vi "cRio_JKS_v5.vi"() -> ()   [LabVIEW 2017]
uses:
  <vilib>/LabVIEW Targets/FPGA/cRIO/shared/nicrio_ModuleControls/nicrio_cRIO-9237_ExcitationVoltageRing.ctl
  <vilib>/LabVIEW Targets/FPGA/cRIO/shared/nicrio_ModuleControls/nicrio_cRIO-9237_DataRatesRing.ctl
  <vilib>/Platform/TimedLoop/XDataNode/timing_clust.ctl
  <vilib>/Platform/TimedLoop/XDataNode/nitl_modes.ctl
  <vilib>/Platform/TimedLoop/XDataNode/wakeup.ctl
  <vilib>/Analysis/3filter.llb/Filter Passband Type.ctl
  <vilib>/rvi/Analysis/host/Butterworth/config/Butterworth Filter Order.ctl
  <vilib>/rvi/Analysis/host/Butterworth/config/Butterworth Filter Type.ctl
  <vilib>/Simulation/Scripting/Companion Diagram/SimConfigNode/SimParams.ctl
  <vilib>/Simulation/Scripting/Companion Diagram/SimConfigNode/_simSolvers.ctl
  <vilib>/Simulation/Implementation/Shared/SIMSCR Execution Mode.ctl
  <vilib>/Simulation/Param Hierarchy/Typedefs/SIMPH Param Control Actions.ctl
  <vilib>/Simulation/Implementation/Shared/NILVSim_ParamChanged.vi
  <vilib>/Simulation/Implementation/Shared/NILVSIM_BeginStep.vi
  <vilib>/Simulation/Implementation/Shared/NILVSim_Manager.vi
  <vilib>/Utility/error.llb/Clear Errors.vi
  <vilib>/Simulation/Implementation/Shared/NILVSim_FinalizeModel.vi
  <vilib>/FPGAPlugInAG/cRIO-9111/niLvFpga_Open_cRIO-9111.vi
  <vilib>/rvi/interface/common/dynamic/niFpgaDynamicAddResources.vi
  <vilib>/rvi/Analysis/host/Butterworth/config/BwScaledCoefficients.vi
  <vilib>/Utility/error.llb/Error Cluster From Error Code.vi
  <vilib>/rvi/errors/niLvFpgaAdjustHostInterfaceError.vi
  <vilib>/Simulation/Implementation/Shared/SIM Unbundle Sim Info.vi
  <vilib>/Simulation/Implementation/Shared/NILVSim_Initialize.vi
  <vilib>/Simulation/Utility/Implementation/NILVSim Get Time and IsAcceptedStep.vi
  <vilib>/Simulation/Implementation/Shared/SIMSH Read Queue.vi
  <vilib>/Simulation/Implementation/Shared/NILVSim_GetModelError.vi
  <vilib>/Simulation/Implementation/Shared/SIM Bundle Sim Info.vi
  <vilib>/FPGAPlugInAG/Dynamic/niLvFpga_Close_Dynamic.vi
  <vilib>/Platform/TimedLoop/XDataNode/XDataNode.xnode
  <vilib>/rvi/interface/nirviOpenFPGA/nirviOpenFPGA.xnode
  FPGA Bitfiles/testrigv1_FPGATarget2_FPGAv3_Z7WGzOqu7JU.lvbitx
  FPGA_JKS_v1.vi
  <vilib>/rvi/Analysis/host/Butterworth/XNode/ButterworthCoefficients.xnode
  <vilib>/rvi/interface/nirviReadWriteControl/nirviReadWriteControl.xnode
  <vilib>/Simulation/Implementation/XNodeFramework/SimXNode/SimX.xnode
  PID (Parallel) with monitoring.vi
  <vilib>/Simulation/Scripting/Companion Diagram/SimConfigNode/SimDog.xnode
  <vilib>/rvi/interface/nirviCloseFPGA/nirviCloseFPGA.xnode
  <vilib>/Platform/TimedLoop/XDataNode/XDNodeRunTimeDep.lvlib
  <vilib>/rvi/interface/Simulation/niFpgaSimulationCallBeginRW.vi
  <vilib>/rvi/Analysis/host/Public/NI_FpgaMspHost.lvlib
  <vilib>/Analysis/NI_AALBase.lvlib
  <vilib>/ptbypt/NI_PtbyPt.lvlib
  NiFpgaLv.dll
  <vilib>/Simulation/Implementation/Shared/NI_SIM_Implementation.lvlib
panel:
  in  "Data Rate Strain Gauge":T1=1 items=["50.000 kS/s (NI 9237)"=1, "25.000 kS/s (NI 9237)"=2, "16.667 kS/s (NI 9237)"=3, "12.500 kS/s (NI 9237)"=4, "10.000 kS/s (NI 9237)"=5, "8.333 kS/s (NI 9237)"=6, "7.143 kS/s (NI 9237)"=7, "6.250 kS/s (NI 9237)"=8, "5.556 kS/s (NI 9237)"=9, "5.000 kS/s (NI 9237)"=10, "4.545 kS/s (NI 9237)"=11, "4.167 kS/s (NI 9237)"=12, "3.846 kS/s (NI 9237)"=13, "3.571 kS/s (NI 9237)"=14, "3.333 kS/s (NI 9237)"=15, "3.125 kS/s (NI 9237)"=16, "2.941 kS/s (NI 9237)"=17, "2.778 kS/s (NI 9237)"=18, "2.632 kS/s (NI 9237)"=19, "2.500 kS/s (NI 9237)"=20, "2.381 kS/s (NI 9237)"=21, "2.273 kS/s (NI 9237)"=22, "2.174 kS/s (NI 9237)"=23, "2.083 kS/s (NI 9237)"=24, "2.000 kS/s (NI 9237)"=25, "1.923 kS/s (NI 9237)"=26, "1.852 kS/s (NI 9237)"=27, "1.786 kS/s (NI 9237)"=28, "1.724 kS/s (NI 9237)"=29, "1.667 kS/s (NI 9237)"=30, "1.613 kS/s (NI 9237)"=31]
  in  "Excitation Voltage Strain Gauge":T2 items=["2.5 Volts", "3.3 Volts", "5.0 Volts", "10.0 Volts", "External Excitation"]
  in  "dpOpen (bar)":sgl=1.0
  out "Run_time slow":dbl
  out "actual_FPGA_dt_(uSec)":u32=50
  out "Actual loop time (mSec)":u32=10
  out "Active.log":bool
  in  "Start.log":bool
  out "P.B.HP":dbl format="%0.2f"
  out "P.B":dbl
  out "P.A1":dbl
  out "P.A":dbl
  out "P.comp":dbl
  out "P.return":dbl
  out "P.pump":dbl
  out "Q.B":dbl format="%0.2f"
  out "FB.Bosch":dbl format="%0.2f"
  out "FB.DCV":dbl format="%0.2f"
  out "u_Bosch":dbl
  out "x.c":dbl
  out "P.B.LP":dbl format="%0.2f"
  out "x.c.dot":dbl
  out "dLcyl filtered":dbl format="%0.2f"
  out "dt":dbl
  in  "Tab Control":enum32{"Settings", "DCV", "Bosch", "ROD"}(tab)
  in  "Bosch mapping 200bar - opening based":cluster{dbl, dbl}[](array[cluster])=[{7.0, 0.0103}, {11.2, 0.032}, {22.0, 0.0535}, {37.0, 0.087}, {61.0, 0.187}, {78.0, 0.289}]
  out "tau (dL)":dbl
  in  "offset_Q_B[V]":sgl=-0.0121
  out "tau (P.B.HP)":dbl
  out "tau (P.B.LP)":dbl
  out "Actual loop time (mSec) slow":u32=10
  in  "Loop time high priority[ms]":i64=10
  in  "cutoff frequency (Hz) FB_Hawe":dbl=300.0
  in  "sample rate (S/s) FB_Hawe":dbl=50000.0
  in  "cutoff frequency (Hz) FB_Bosch":dbl=1000.0
  in  "sample rate (S/s) FB_Bosch":dbl=50000.0
  in  "cutoff frequency (Hz) FB_PVG":dbl=1000.0
  in  "sample rate (S/s) FB_PVG":dbl=50000.0
  in  "cutoff frequency (Hz) Q":dbl=50.0
  in  "sample rate (S/s) Q":dbl=50000.0
  in  "sample rate (S/s) l_cyl":dbl=50000.0
  in  "cutoff frequency (Hz)l_cyl":dbl=400.0
  in  "sample rate (S/s) pressures":dbl=50000.0
  in  "cutoff frequency (Hz) pressures":dbl=100.0
  out "FPGA_dt(uSec) slow":u32=50
  in  "FPGA_dt(uSec)":u32=50
  in  "dL lowpass cutoff freq [Hz]":dbl=8.0 format="%0.3f"
  in  "Initialise dL lowpass filter":bool
  in  "dL HP cutoff freq [Hz]":dbl=2.5
  out "tau (dL) slow":dbl
  in  "Pb highpass cutoff freq [Hz]":dbl=1.411 format="%0.3f"
  in  "Initialise Pb highpass filter":bool
  in  "Pb lowpass cutoff freq [Hz]":dbl=0.5 format="%0.3f"
  in  "Initialise Pb lowpass filter":bool
  out "tau (P.B.HP) slow":dbl
  out "tau (P.B.LP) slow":dbl
  in  "Bosch mapping 200bar - average based":cluster{dbl, dbl}[](array[cluster])=[{7.0, 0.0103}, {12.5, 0.032}, {24.0, 0.0535}, {38.5, 0.087}, {63.3, 0.187}, {80.0, 0.289}]
  in  "Bosch mapping 180bar - opening based":cluster{dbl, dbl}[](array[cluster])=[{4.0, 0.0103}, {8.3, 0.032}, {17.0, 0.053}, {29.0, 0.087}, {51.0, 0.187}, {80.0, 0.38}]
  in  "cutoff frequency (Hz) Strain":dbl=100.0
  in  "sample rate (S/s) Strain":dbl=50000.0
  in  "DCV Input type":i32(listbox)
  in  "Valve limit positioning [u]":dbl=0.2
  in  "Kp.pos.cyl1":dbl=3.0
  in  "Wanted cylinder position [m]":dbl=0.42 step=0.1
  out "Active - Cylinder 1 positioning":bool
  in  "Start control cylinder 1":bool
  in  "Activate DCV":bool=TRUE
  in  "DCV Output":i32(listbox)
  in  "Activate comp":bool
  in  "Comp.Q.to.U.gain":dbl=2401.15
  in  "Comp.kF.gain":dbl=3e-06
  in  "Start log with ramp":bool
  in  "Direction":bool
  out "Ramp array":dbl[][](array[numeric])
  out "Ramp elapsed time":dbl
  out "Ramp active":bool
  in  "Activate ramp":bool
  in  "Ramp ymax":dbl=0.15
  in  "Ramp t_ramp [s]":dbl=8.0
  in  "Ramp tr [s]":dbl=1.0
  in  "Ramp td [s]":dbl=1.0
  in  "Reset":bool
  in  "DCV, setpoint (slider)":dbl(slide) min=-1.0 max=1.0 step=0.05 scale=0.5..-0.5
  out "Ramp active VIDEO":bool
  out "Motion VIDEO":bool
  in  "Bosch input type":i32(listbox)
  in  "Activate Bosch":bool
  in  "Reset Bosch":bool
  in  "Bosch valve, voltage":dbl(slide) min=-1.0 max=1.0 step=0.05 scale=0.0..1.0
  in  "Start log with ramp 2":bool
  in  "Start - Bosch array":bool
  in  "Bosch array":cluster{dbl, dbl}[](array[cluster])=[{0.0, 0.0}, {15.0, 0.45}, {17.0, 0.45}, {32.0, 0.0}]
  out "Elapsed time 2":dbl
  in  "Start log with ramp 3":bool
  in  "Start - Bosch Fake PB":bool
  in  "Bosch array 2":cluster{dbl, dbl}[](array[cluster])=[{0.0, 5.0}, {0.01, 40.0}, {4.0, 40.0}, {4.01, 5.0}, {8.0, 5.0}, {9.0, 5.0}]
  out "Elapsed time 3":dbl
  in  "Activate limits":bool
  in  "Upper pressure limit [bar]":dbl=75.0 format="%#_13g"
  in  "Lower pressure limit [bar]":dbl=4.0 format="%#_13g"
  in  "Bypass low-pass filter":bool
  in  "Fake pressure type":i32(listbox)
  in  "Fake p.comp slider":dbl(slide) min=-1.0 max=1.0 step=0.05 scale=0.0..200.0
  in  "Feed forward activate":bool
  in  "Derivative Gain 2":dbl
  in  "Integral Gain 2":dbl=0.0012
  in  "Proportional Gain 2":dbl=0.005
  in  "Controller selection":i32(listbox)
  in  "Derivative Gain":dbl
  in  "Integral Gain":dbl=0.004
  in  "Proportional Gain":dbl=0.001
  in  "Initialize bosch":bool
  in  "Reset Bosch 2":bool
  in  "Bosch valve, pressure":dbl(slide) min=-1.0 max=1.0 step=0.05 scale=0.0..150.0
  in  "Run Bosch control system":bool
  in  "Operation mode":bool
  out "Run_time":dbl
  out "u_DCV_comp":dbl
  out "u_DCV":dbl
  out "U_PVG":sgl=6.0
  out "U_Bosch":sgl
  out "U_Hawe":sgl
  # "Active"
  # "SENSOR OFFEST AND VOLTAGE CONTROL"
  # "cRIO LOOP CONTROL"
  # "FPGA FILTER CONTROL"
  # "Pressure sensors"
  # "DCV feedback sensors"
  # "Cylinder position sensor"
  # "Flow sensor"
  # "PRV feedback sensor"
  # "FPGA LOOP CONTROL"
  # "Cylinder filters"
  # "tau = 0,1 er et godt startgæt"
  # "Pressure filters"
  # "Position controller"
  # "[0 ... 0,5]"
  # "Pressure feedback Compensation"
  # "RAMP CONTROL"
  # "UP"
  # "DOWN"
  # "MANUAL CONTROL"
  # "UP"
  # "DOWN"
  # "MANUAL CONTROL"
  # "CLOSE"
  # "(Increase\nPressure)"
  # "OPEN"
  # "(Decrease\nPressure)"
  # "Array direct control"
  # "CONTROL SYSTEM"
  # "AUTO MODE"
  # "Fake PB array"
  # "PRESSURE LIMITS"
  # "FAKE PB PRESSURE"
  # "CONTROLLER SETTINGS"
  # "Controller 1"
  # "Controller 2"
  # "MANUAL PRESSURE CONTROL (no filter)"
  # "HIGH"
  # "LOW"
  # "RAMP CONTROL"
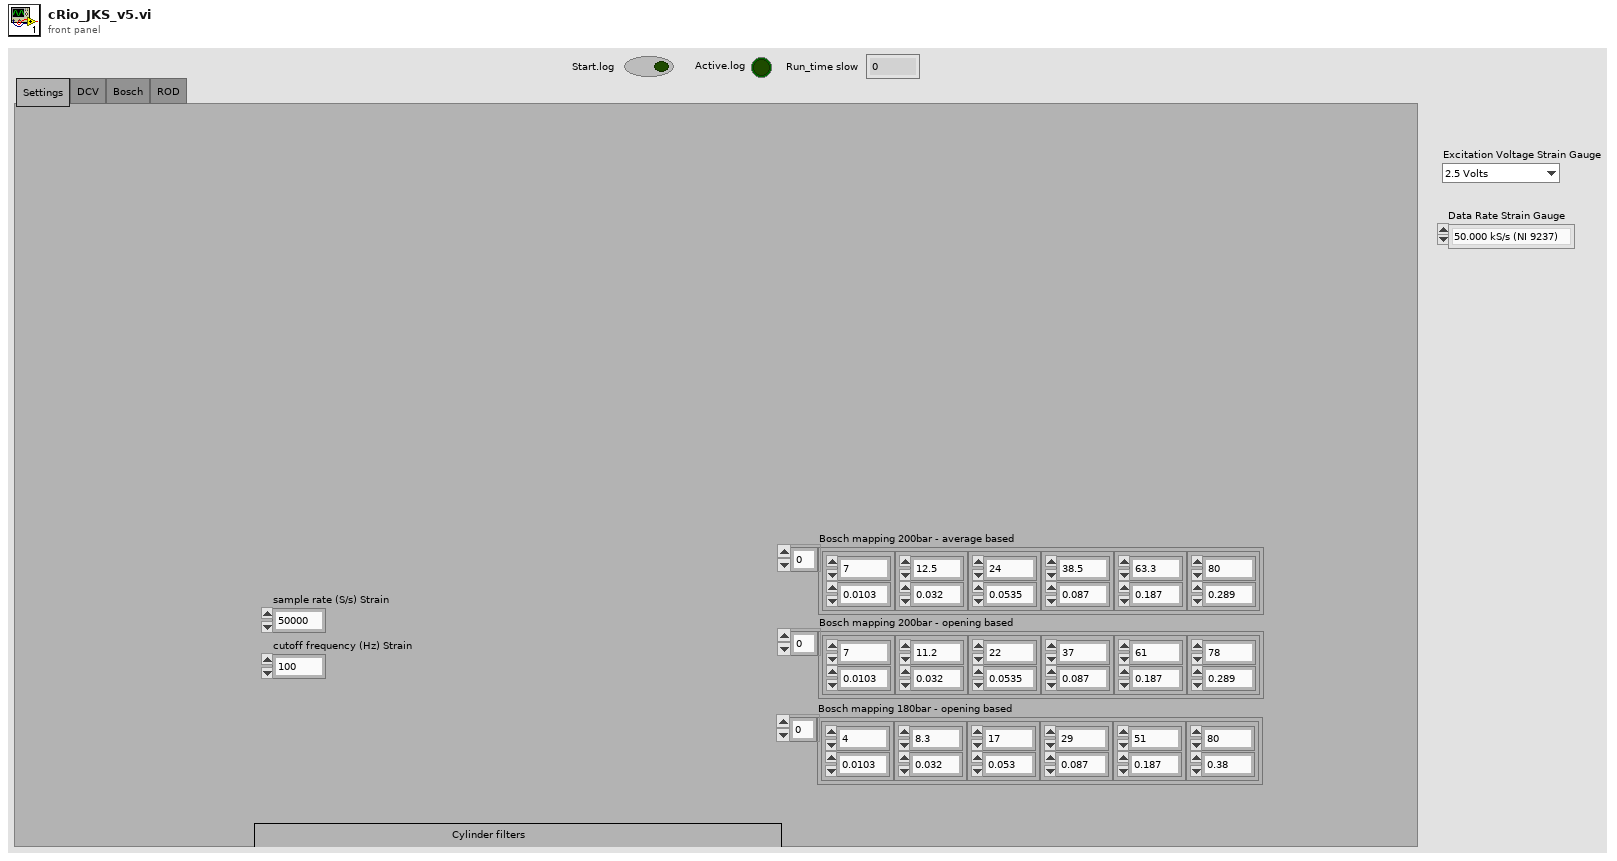
[diagram p1: front panel]
types:
  T1 = typedef "nicrio_cRIO-9237_DataRatesRing.ctl" = u8
  T2 = typedef "nicrio_cRIO-9237_ExcitationVoltageRing.ctl" = u8
  T3 = typedef "XDNodeRunTimeDep.lvlib/timing_clust.ctl" = cluster{"Expected End [f-1]":u64, "Actual End [f-1]":u64, "Finished Late? [f-1]":bool, "Expected End [i-1]":u64, "Actual End [i-1]":u64, "Finished Late? [i-1]":bool, "Expected Start [i]":u64, "Actual Start [i]":u64, "Expected Start [f]":u64, "Actual Start [f]":u64, "Source Name":string, "Structure Name":string, "Period":i64, "Deadline":i64, "Offset":i64, "Start":i64, "Priority":i32, "Timeout":i32, "Mode":T4, "Wakeup Reason":T5, "Error":errorcluster, "Source Type":string, "Secondary Source Type":string, "Global End Time":u64, "Global Start Time":u64, "Frame Duration":u64, "Iteration Duration":u64, "Assigned CPU":i32, "I/O Scan Engine Mode":u32}
  T4 = typedef "XDNodeRunTimeDep.lvlib/nitl_modes.ctl" = enum32{"No Change", "Process missed periods, maintain original phase", "Discard missed periods, maintain original phase", "Process missed periods, ignore original phase", "Discard missed periods, ignore original phase"}
  T5 = typedef "XDNodeRunTimeDep.lvlib/wakeup.ctl" = enum32{"Normal", "Aborted", "Asynchronous wakeup", "Timing source error", "Timed loop error", "Timeout"}
  T6 = typedef "NI_AALBase.lvlib/Filter Passband Type.ctl" = enum32{"Lowpass", "Highpass", "Bandpass", "Bandstop"}
  T7 = enum16{"Simulate to Completion", "Single Time-Step Simulation (Fixed Step Only)"}
  T8 = typedef "SIMSCR Execution Mode.ctl" = enum16{"Simulate to Completion", "Single Time-Step Simulation (Fixed Step Only)"}
  T9 = typedef "SIMPH Param Control Actions.ctl" = enum16{"get params", "set params"}
  T10 = cluster{"SIMSH Sim Time":dbl, "Build Array":cluster{"appended array":dbl[]}, "Integral Gain - series.vi":cluster{"output":dbl}, "Integral Gain - series.vi - SIMSH":cluster{"SIMSH Sim Time":dbl, "Select 2":cluster{"s? t:f":dbl}, "integral in gain?":bool, "Integrator":cluster{"output y(t)":dbl}, "Gain 2":cluster{"output":dbl}, "Select":cluster{"s? t:f":dbl}, "Equal To 0?":cluster{"x = 0?":bool}, "Reciprocal":cluster{"1/x":dbl}}, "SIM PID Derivative Gain.vi":cluster{"output":dbl}, "SIM PID Derivative Gain.vi - SIMSH":cluster{"SIMSH Sim Time":dbl, "t 3":dbl, "Select 2":cluster{"s? t:f":dbl}, "Equal?":cluster{"x = y?":bool}, "Or":cluster{"x .or. y?":bool}, "Equal To 0?":cluster{"x = 0?":bool}}, "Gain":cluster{"output":dbl}, "Summation":cluster{"Result":dbl}}
  T11 = typedef "SimParams.ctl" = cluster{"Initial Time (s)":dbl, "Final Time (s)":dbl, "Step Size (s)":dbl, "ODE Solver":T12, "Minimum Step Size (s)":dbl, "Maximum Step Size (s)":dbl, "Relative Tolerance":dbl, "Absolute Tolerance":dbl, "Software Timing":bool, "Initial Step Size (s)":dbl, "Automatic Fixed Step Size?":bool, "Automatic Discrete Step Size?":bool, "Discrete Step Size (s)":dbl, "Calculate using Time Step":bool, "Solver Wired?":bool, "Prev.Frm.Expected End":u64, "Prev.Frm.Actual End":u64, "Prev.Frm.Finished Late?":bool, "Prev.Iter.Expected End":u64, "Prev.Iter.Actual End":u64, "Prev.Iter.Finished Late?":bool, "Expected Iteration Start":u64, "Actual Iteration Start":u64, "Expected Frame Start":u64, "Actual Frame Start":u64, "Source Name":string, "Name":string, "Period":i64, "Deadline":i64, "Offset":i64, "Start":i64, "Priority":i32, "Timeout":i32, "Processor":i32, "Mode":enum32{"No Change", "Process missed periods, maintain original phase", "Discard missed periods, maintain original phase", "Process missed periods, ignore original phase", "Discard missed periods, ignore original phase"}, "Wakeup reason":enum32{"Normal", "Aborted", "Asynchronous wakeup", "Timing source error", "Timed loop error", "Timeout"}, "Error":errorcluster, "Source Type":string, "Secondary Source Type":string, "Global End Time":u64, "Global Start Time":u64, "Full Solver Reset":bool, "Execution Mode":T8, "Nan/Inf Check":bool, "Custom Solver Library":string, "Solver Is Variable":bool, "custom solver name":string, "Signal Collection Decimation":u32}
  T12 = typedef "_simSolvers.ctl" = enum16{"Runge-Kutta 1 (Euler)", "Runge-Kutta 2", "Runge-Kutta 3", "Runge-Kutta 4", "Runge-Kutta 23 (variable)", "Runge-Kutta 45 (variable)", "BDF (variable)", "Adams-Moulton (variable)", "Rosenbrock (variable)", "Discrete States Only", "SDIRK 4 (variable)", "Radau 5 (variable)", "Radau 9 (variable)", "Radau 13 (variable)", "Radau [Variable Order] (variable)", "Gear's Method (variable)", "Linearizer", "State Query", "Trim Eval", "Custom Solver"}
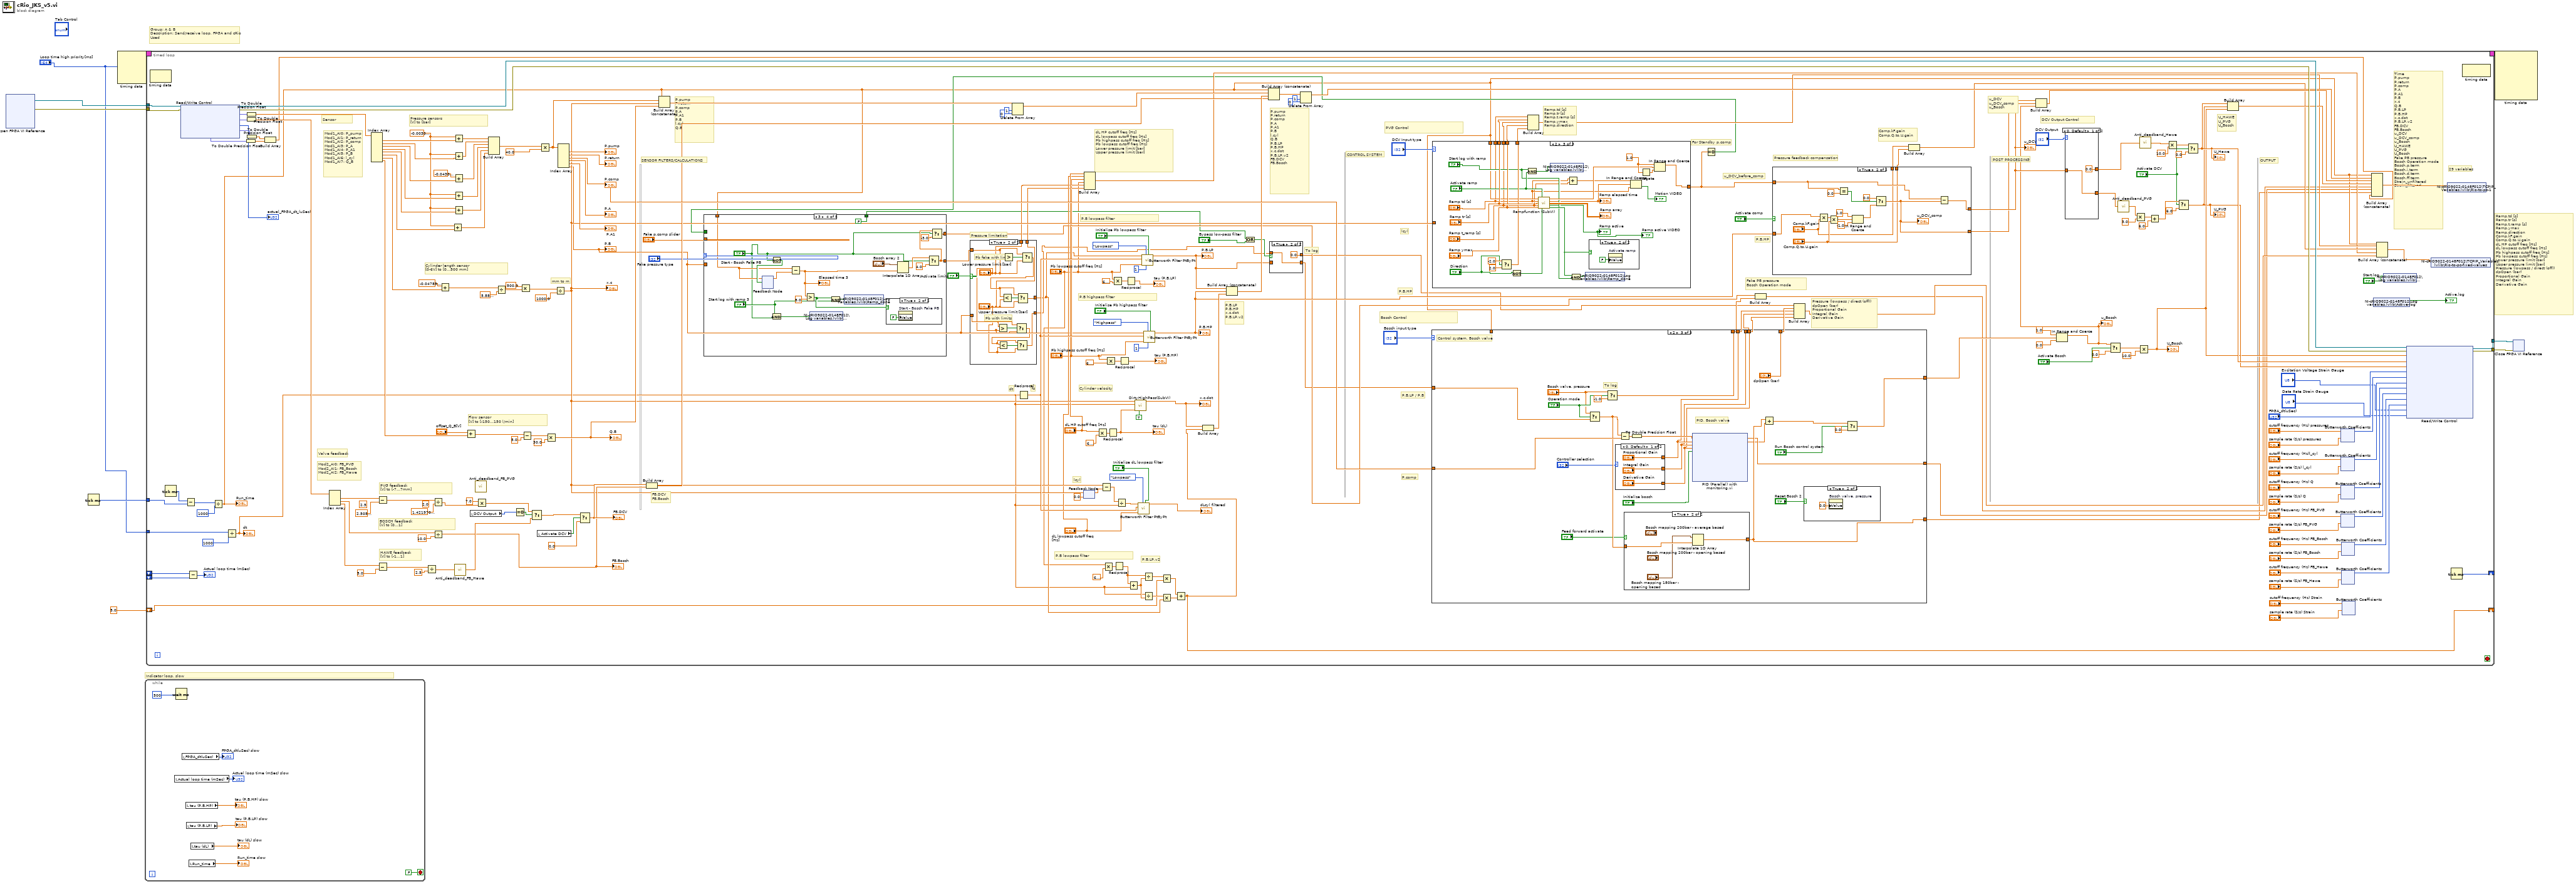
[diagram p0: block diagram]
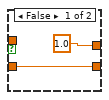
[diagram p2: hidden frame]
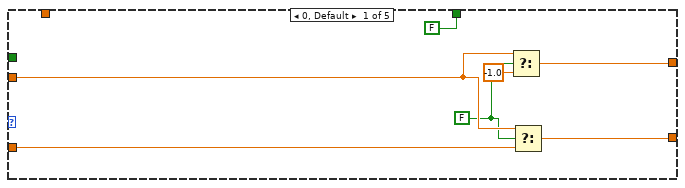
[diagram p3: hidden frame]
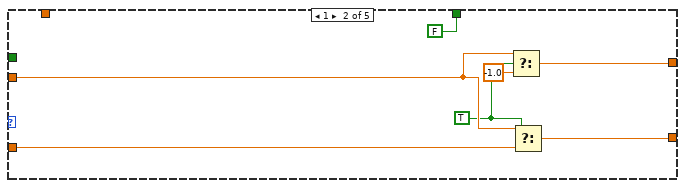
[diagram p4: hidden frame]
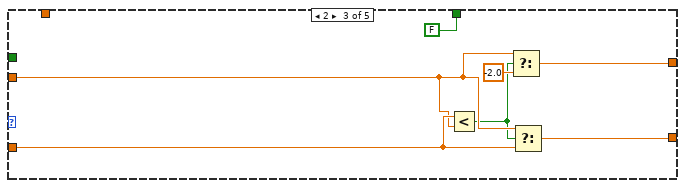
[diagram p5: hidden frame]
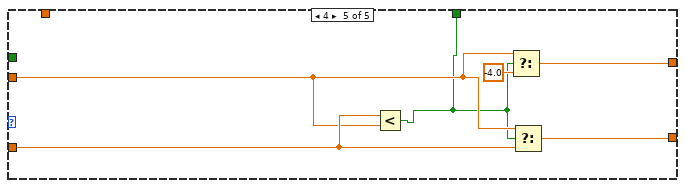
[diagram p7: hidden frame]
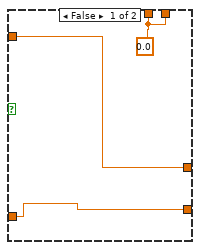
[diagram p8: hidden frame]
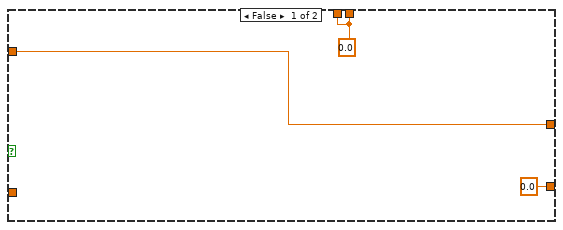
[diagram p9: hidden frame]
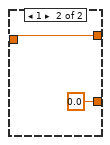
[diagram p10: hidden frame]
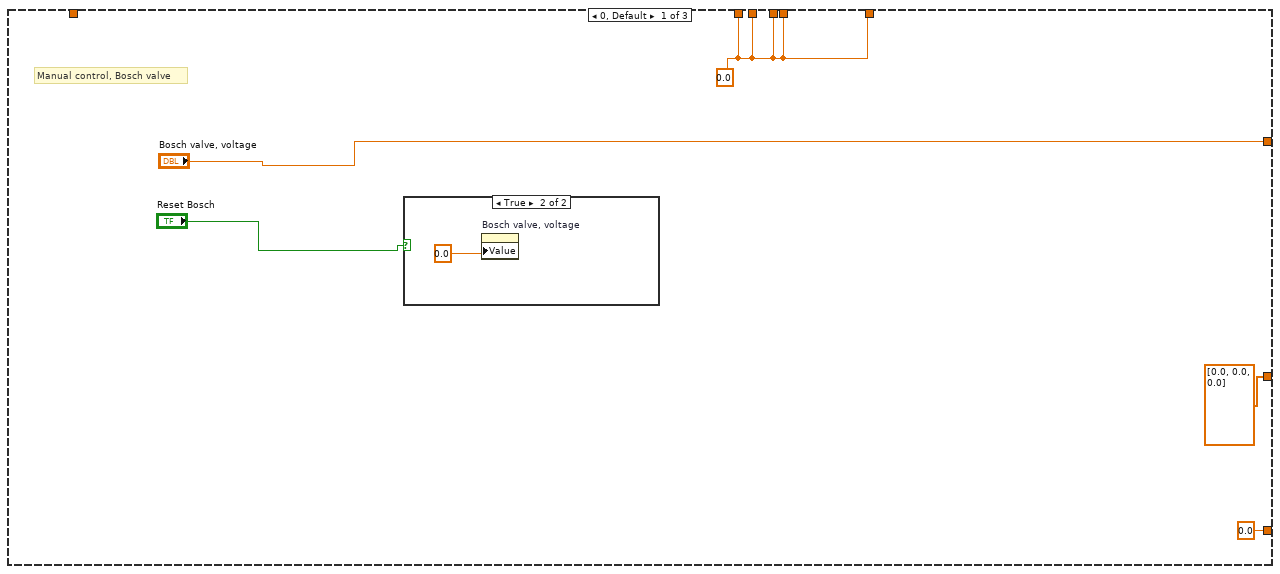
[diagram p11: hidden frame]
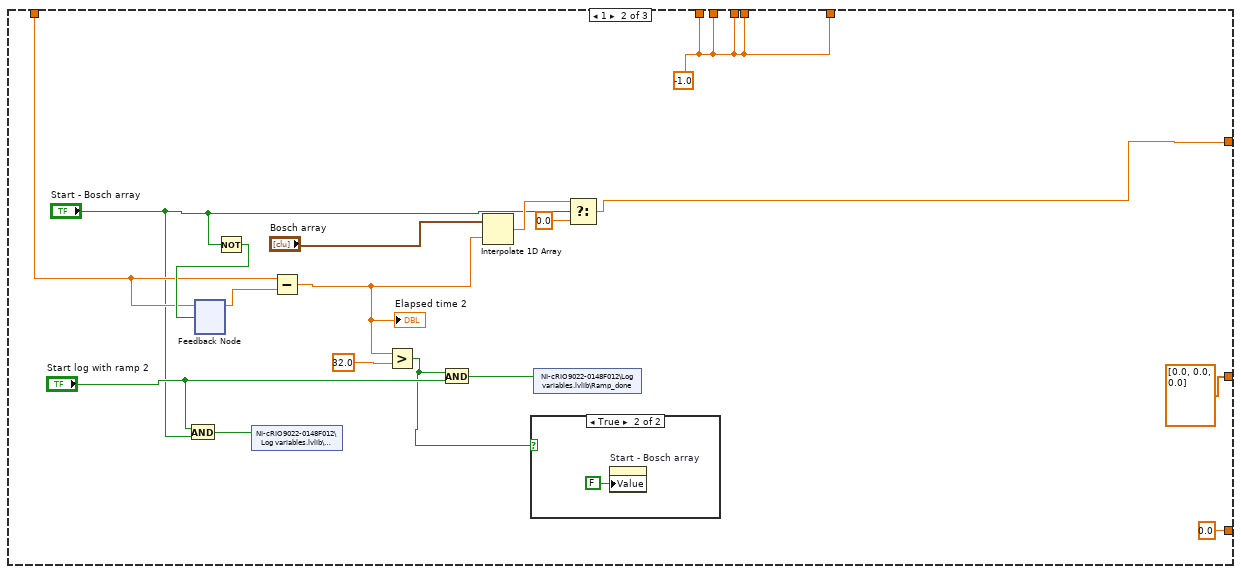
[diagram p13: hidden frame]
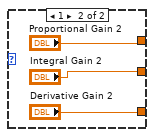
[diagram p15: hidden frame]
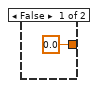
[diagram p16: hidden frame]
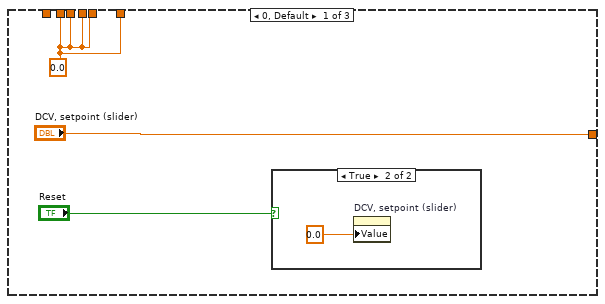
[diagram p18: hidden frame]
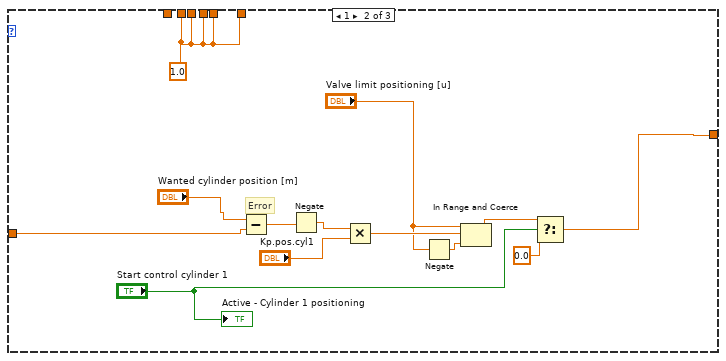
[diagram p20: hidden frame]
diagram:
  # "Ramp.td [s]\nRamp.tr [s]\nRamp.t.ramp [s]\nRamp.ymax\nRamp.direction\nComp.kF.gain\nComp.Q.to.U.gain\ndL HP cutoff freq [Hz]\ndL lowpass cutoff freq [Hz]\nPb highpass cutoff freq [Hz]\nPb lowpass cutoff freq [Hz]\nLower pressure limit [bar]\nUpper pressure limit [bar]\nPressure (lowpass / direct (off))\ndpOpen (bar)\nProportional Gain\nIntegral Gain\nDerivative Gain"
  # "Indicator loop, slow"
  # "Group: A & B\nDescription: Send/receive loop, FPGA and cRio\nUsed"
  n1 = xnode "Open FPGA VI Reference"() -> ("FPGA VI Reference Out"=w7:refnum<k20>, "error out"=w6:errorcluster)  [unwired: 2 in]
  n2 = Tick Count (ms)() -> (millisecond timer value=w3:u32)
  n3 = node-c288("Loop time high priority[ms]") -> (w9:T3)  [unwired: 3 in]
  n4 = while {
    stop <- FALSE stop-if-true
    n5 = local read "Actual loop time (mSec)"() -> (→"Actual loop time (mSec) slow":u32)
    n6 = Wait (ms)(milliseconds to wait=i64 500 ("Period")) -> ()  [unwired: 1 out]
    n7 = local read "FPGA_dt(uSec)"() -> (→"FPGA_dt(uSec) slow":u32)
    n8 = local read "tau (P.B.HP)"() -> (→"tau (P.B.HP) slow":dbl)
    n9 = local read "tau (P.B.LP)"() -> (→"tau (P.B.LP) slow":dbl)
    n10 = local read "Run_time"() -> (→"Run_time slow":dbl)
    n11 = local read "tau (dL)"() -> (→"tau (dL) slow":dbl)
  }
  n12 = timed-loop {
    timing: w9 -> [_]
    timing-out: [_] -> w8
    tunnel: w7 -> [w175]
    tunnel: w6 -> [w174]
    tunnel: [w171] -> w5
    tunnel: [w170] -> w4
    tunnel: w3 -> [w160]
    shift-right: [w164] -> _
    shift-left: _ -> [w163]
    shift-left: _ -> [w162]
    tunnel: "Loop time high priority[ms]" -> [w159]
    shift-right: [w27] -> _
    shift-left: 5.0 -> [w29]
    stop <- _ stop-if-true
    w180 = sgl -0.003 ("x")
    (unwired) sgl 2.0 ("y")
    (unwired) sgl 2.5 ("y")
    # "P.B lowpass filter"
    # "P.B.LP.v2"
    # "To log"
    # "For Standby p.comp"
    # "Fake PB pressure\nBosch Operation mode"
    # "Pressure (lowpass / direct (off))\ndpOpen (bar)\nProportional Gain\nIntegral Gain\nDerivative Gain"
    # "Pressure limitation"
    # "dL HP cutoff freq [Hz]\ndL lowpass cutoff freq [Hz]\nPb highpass cutoff freq [Hz]\nPb lowpass cutoff freq [Hz]\nLower pressure limit [bar]\nUpper pressure limit [bar]"
    # "mm to m"
    # "29 variables"
    # "Comp.kF.gain\nComp.Q.to.U.gain"
    # "Time\nP.pump\nP.return\nP.comp\nP.A\nP.A1\nP.B\nx.c\nQ.B\nP.B.LP\nP.B.HP\nx.c.dot\nP.B.LP.v2\nFB.DCV\nFB.Bosch\nu_DCV\nu_DCV_comp\nu_Bosch\nU_HAWE\nU_PVG\nU_Bosch\nFake PB pressure\nBosch Operation mode\nBosch.p.term\nBosch.i.term\nBosch.d.term\nBosch.ff.term\nStrain_unfiltered\nStrain_filtered"
    # "u_DCV_before_comp"
    # "P.B.HP"
    # "SENSOR FILTERS/CALCULATIONS"
    # "CONTROL SYSTEM"
    # "P.B highpass filter"
    # "FB.DCV\nFB.Bosch"
    # "P.B.LP\nP.B.HP\nx.c.dot\nP.B.LP.v2"
    # "P.pump\nP.return\nP.comp\nP.A\nP.A1\nP.B\nl.cyl\nQ.B"
    # "P.pump\nP.return\nP.comp\nP.A\nP.A1\nP.B\nl.cyl\nQ.B\nP.B.LP\nP.B.HP\nx.c.dot\nP.B.LP.v2\nFB.DCV\nFB.Bosch"
    # "fs"
    # "lcyl"
    # "P.B.HP"
    # "lcyl"
    # "POST PROCESSING"
    # "OUTPUT"
    # "Ramp.td [s]\nRamp.tr [s]\nRamp.t.ramp [s]\nRamp.ymax\nRamp.direction"
    # "u_DCV\nu_DCV_comp\nu_Bosch"
    # "U_HAWE\nU_PVG\nU_Bosch"
    # "DCV Output Control"
    # "Bosch Control"
    # "Pressure feedback compensation"
    # "P.comp"
    # "P.B.LP / P.B"
    # "dt"
    # "Cylinder velocity"
    # "P.B lowpass filter"
    # "PVG Control"
    # "Cylinder length sensor\n[0-6V] to [0...500 mm]"
    # "Flow sensor\n[V] to [-150...150 l/min]"
    # "BOSCH feedback\n[V] to [0...1]"
    # "HAWE feedback\n[V] to [-1...1]"
    # "PVG feedback\n[V] to [-7...7mm]"
    # "Pressure sensors\n[V] to [bar]"
    # "Valve feedback"
    # "Mod2_AI0: FB_PVG\nMod2_AI1: FB_Bosch\nMod2_AI2: FB_Hawe"
    # "Sensor"
    # "Mod1_AI0: P_pump\nMod1_AI1: P_return\nMod1_AI2: P_comp\nMod1_AI3: P_A\nMod1_AI4: P_A1\nMod1_AI5: P_B\nMod1_AI6: l_cyl\nMod1_AI7: Q_B"
    n13 = node-c288() -> ()  [unwired: 1 in, 1 out]
    n14 = Tick Count (ms)() -> (millisecond timer value=w166:u32)
    n15 = xnode "Read/Write Control"("FPGA VI Reference In"=w175, "error in"=w174) -> ("FPGA VI Reference Out"=w173:refnum<k20>, "error out"=w172:errorcluster, "all_sensors"=w250:fxp<+/-,24,13>[], "FB_valves"=w220:fxp<+/-,20,9>[], "actual_FPGA_filter_dt(uSec)"=→"actual_FPGA_dt_(uSec)":u32, "Strain_unfiltered"=w26:fxp<+/-,24,3>, "Strain_filtered"=w25:fxp<+/-,24,3>)
    n16 = Subtract(x=w166, y=w160) -> (x-y=w168:u32)
    n17 = Subtract(x=w163, y=w162) -> (x-y=→"Actual loop time (mSec)":u32)
    n18 = Divide(x=w168, y=u32 1000) -> (x/y=w52:dbl)
    "Run_time" <- w52
    n19 = Divide(x=w159, y=u32 1000) -> (x/y=w31:dbl)
    "dt" <- w31
    n20 = To Double Precision Float(number=w25) -> (double precision float=w21:dbl)
    n21 = To Double Precision Float(number=w250) -> (double precision float=w249:dbl[])
    n22 = To Double Precision Float(number=w220) -> (double precision float=w211:dbl[])
    n23 = To Double Precision Float(number=w26) -> (double precision float=w22:dbl)
    n24 = Build Array(w22, w21) -> (w20:dbl[])
    n25 = Index Array(array=w211) -> (element #1=w179:dbl, element #2=w188:dbl, element #3=w194:dbl)  [unwired: 3 in]
    n26 = Index Array(array=w249) -> (element #1=w232:dbl, element #2=w176:dbl, element #3=w230:dbl, element #4=w229:dbl, element #5=w228:dbl, element #6=w227:dbl, element #7=w226:dbl, element #8=w225:dbl)  [unwired: 8 in]
    n27 = Subtract(x=w179, y=sgl 2.505) -> (x-y=w241:dbl)
    n28 = Subtract(x=w194, y=sgl 5.0) -> (x-y=w192:dbl)
    n29 = Divide(x=w192, y=sgl 2.5) -> (x/y=w195:dbl)
    n30 = Divide(x=w241, y=sgl 1.42197) -> (x/y=w55:dbl)
    n31 = Divide(x=w188, y=sgl 10.0) -> (x/y=w111:dbl)
    "FB.Bosch" <- w111
    n32 = Add(x=sgl -0.0479, y=w226) -> (x+y=w234:dbl)
    n33 = Add(x=w180, y=w227) -> (x+y=w141:dbl)
    n34 = Add(x=w180, y=w232) -> (x+y=w231:dbl)
    n35 = Add(x=w180, y=w176) -> (x+y=w245:dbl)
    n36 = Add(x=sgl -0.043, y=w230) -> (x+y=w140:dbl)
    n37 = Add(x=w180, y=w229) -> (x+y=w244:dbl)
    n38 = Add(x=w180, y=w228) -> (x+y=w243:dbl)
    n39 = call "Anti_deadband_FB_Hawe.vi"("x"=w195) -> ("y"=w177:sgl)
    n40 = Add(x="offset_Q_B[V]", y=w225) -> (x+y=w235:dbl)
    n41 = local read "DCV Output"() -> (w131:i32)
    n42 = call "Anti_deadband_FB_PVG.vi"() -> ()  [unwired: 1 in, 1 out]
    n43 = Multiply(x=7.0, y=w55) -> (x*y=w53:dbl)
    n44 = Build Array(w231, w245, w140, w244, w243, w141) -> (w233:dbl[])
    n45 = Divide(x=w234, y=sgl 5.89 ("x")) -> (x/y=w240:dbl)
    n46 = Equal To 0?(x=w131) -> (x = 0?=w130:bool)
    n47 = Multiply(x=sgl 500.0, y=w240) -> (x*y=w80:dbl)
    n48 = Subtract(x=w235, y=sgl 5.0) -> (x-y=w191:dbl)
    n49 = Select(t=w53, s=w130, f=w177) -> (s? t:f=w213:dbl)
    n50 = local read "Activate DCV"() -> (w132:bool)
    n51 = Multiply(x=w233, y=sgl 40.0 ("Mod1/AI5")) -> (x*y=w169:dbl[])
    n52 = Multiply(x=w191, y=sgl 30.0) -> (x*y=w106:dbl)
    "Q.B" <- w106
    n53 = Divide(x=w80, y=sgl 1000.0) -> (x/y=w81:dbl)
    "x.c" <- w81
    n54 = Index Array(array=w169) -> (element #1=→"P.pump":dbl, element #2=→"P.return":dbl, element #3=w101:dbl, element #4=→"P.A":dbl, element #5=→"P.A1":dbl, element #6=w43:dbl)  [unwired: 6 in]
    "P.comp" <- w101
    "P.B" <- w43
    n55 = Select(t=w213, s=w132, f=sgl 0.0) -> (s? t:f=w112:dbl)
    "FB.DCV" <- w112
    n56 = Build Array(w112, w111) -> (w82:dbl[])
    n57 = Build Array (concatenate)(w52, w169, w81, w106) -> (w95:dbl[])
    n58 = Delete From Array(array=w95, length=1, index=0) -> (array with subset deleted=w94:dbl[])  [unwired: 1 out]
    n59 = Reciprocal(x=w31) -> (1/x=w104:dbl)
    n60 = feedback #1(sgl 0.0 ("Single")) -> (w155:dbl)
    n61 = feedback-in #1(w81) -> ()
    n62 = Multiply(x="dL HP cutoff freq [Hz]", y=sgl 6.2831855) -> (x*y=w151:dbl)
    n63 = Subtract(x=w81, y=w155) -> (x-y=w149:dbl)
    n64 = Multiply(x="Pb lowpass cutoff freq [Hz]", y=sgl 6.2831855) -> (x*y=w34:dbl)
    n65 = Multiply(x="Pb highpass cutoff freq [Hz]", y=sgl 6.2831855) -> (x*y=w114:dbl)
    n66 = Reciprocal(x=w151) -> (1/x=w150:dbl)
    "tau (dL)" <- w150
    n67 = Multiply(x="Pb lowpass cutoff freq [Hz]", y=sgl 6.2831855) -> (x*y=w138:dbl)
    n68 = Reciprocal(x=w34) -> (1/x=w33:dbl)
    n69 = Divide(x=w149, y=w31) -> (x/y=w145:dbl)
    n70 = Reciprocal(x=w114) -> (1/x=→"tau (P.B.HP)":dbl)
    n71 = Reciprocal(x=w138) -> (1/x=→"tau (P.B.LP)":dbl)
    n72 = Add(x=w33, y=w31) -> (x+y=w38:dbl)
    n73 = call "DirtyHighPass(SubVI).vi"("Enable"=TRUE, "tau"=w150, "dt[s]"=w31, "Numeric in"=w81) -> ("Numeric out"=w146:dbl)  [unwired: 7 in]
    "x.c.dot" <- w146
    n74 = call <vilib>:"Butterworth Filter PtByPt.vi"("initialize"="Initialise dL lowpass filter", "filter type"=Filter_Passband_Type."Lowpass", "low cutoff freq: fl"="dL lowpass cutoff freq [Hz]", "sampling freq: fs"=w104, "x"=w145) -> ("Filtered x"=→"dLcyl filtered":dbl)  [unwired: 4 in, 1 out]
    n75 = Divide(x=w33, y=w38) -> (x/y=w40:dbl)
    n76 = Divide(x=w31, y=w38) -> (x/y=w37:dbl)
    n77 = call <vilib>:"Butterworth Filter PtByPt.vi"("initialize"="Initialise Pb highpass filter", "order"=1, "filter type"=Filter_Passband_Type."Highpass", "low cutoff freq: fl"="Pb highpass cutoff freq [Hz]", "sampling freq: fs"=w104, "x"=w43) -> ("Filtered x"=w102:dbl)  [unwired: 3 in, 1 out]
    "P.B.HP" <- w102
    n78 = Multiply(x=w40, y=w29) -> (x*y=w39:dbl)
    n79 = case shown="2" "DCV Input type" {
      tunnel: w52 -> [_ _ w697]
      tunnel: w81 -> [_ w683 _]
      tunnel: ["DCV, setpoint (slider)" w682 w711] -> w61
      tunnel: [w676 w681 "Ramp td [s]"] -> w123
      tunnel: [w676 w681 "Ramp tr [s]"] -> w122
      tunnel: [w676 w681 "Ramp t_ramp [s]"] -> w121
      tunnel: [w676 w681 "Ramp ymax"] -> w120
      tunnel: [w676 w681 w706] -> w119
      frame 0, Default {
        w676 = 0.0 ("Ramp td [s]")
        n80 = case shown="True" "Reset" {
          frame False {
          }
          frame True {
            n81 = property on="DCV, setpoint (slider)" class="Slide (strict)"("Value"=0.0 ("t")) -> ()  [unwired: 2 in, 2 out]
          }
        }
      }
      frame 1 {
        w681 = 1.0 ("Ramp td [s]")
        # "Error"
        n82 = Subtract(x="Wanted cylinder position [m]", y=w683) -> (x-y=w680:dbl)
        n83 = Negate(x=w680) -> (-x=w679:dbl)
        n84 = Multiply(x=w679, y="Kp.pos.cyl1") -> (x*y=w689:dbl)
        n85 = Negate(x="Valve limit positioning [u]") -> (-x=w690:dbl)
        n86 = In Range and Coerce(upper limit="Valve limit positioning [u]", x=w689, lower limit=w690) -> (coerced(x)=w691:dbl)  [unwired: 1 out]
        n87 = Select(t=w691, s="Start control cylinder 1", f=0.0) -> (s? t:f=w682:dbl)
        "Active - Cylinder 1 positioning" <- "Start control cylinder 1"
      }
      frame 2 {
        w713 = 1.0 ("upper limit")
        n88 = Select(t=-2.0, s="Direction", f=2.0) -> (s? t:f=w706:dbl)
        n89 = Not(x="Direction") -> (.not. x?=w700:bool)
        n90 = And(x="Start log with ramp", y="Activate ramp") -> (x .and. y?=w705:bool)
        n91 = call "Rampfunction (SubVI).vi"("Time"=w697, "Ramp activate"="Activate ramp", "Ramp td [s]"="Ramp td [s]", "Ramp tr [s]"="Ramp tr [s]", "Ramp t_ramp [s]"="Ramp t_ramp [s]", "Ramp ymax"="Ramp ymax", "Direction"=w700) -> ("y"=w712:dbl, "ramp time"=w692:dbl, "Ramp array"=→"Ramp array":dbl[][], "Ramp active"=→"Ramp active" →"Ramp active VIDEO":bool, "Ramp done"=w702:bool)  [unwired: 4 in]
        "Ramp elapsed time" <- w692
        n92 = shared-variable "NI-cRIO9022-0148F012\\Log variables.lvlib\\Start-log"(w705) -> ()  [unwired: 1 in, 1 out]
        n93 = Add(x="Ramp td [s]", y="Ramp t_ramp [s]") -> (x+y=w696:dbl)
        n94 = And(x=w702, y="Start log with ramp") -> (x .and. y?=w703:bool)
        n95 = shared-variable "NI-cRIO9022-0148F012\\Log variables.lvlib\\Ramp_done"(w703) -> ()  [unwired: 1 in, 1 out]
        n96 = case shown="True" w702 {
          frame False {
          }
          frame True {
            n97 = property on="Activate ramp" class="Bool (strict)"("Value"=FALSE ("Activate ramp")) -> ()  [unwired: 2 in, 2 out]
          }
        }
        n98 = In Range and Coerce(upper limit=w696, x=w692, lower limit="Ramp td [s]") -> (In Range?=→"Motion VIDEO":bool)  [unwired: 1 out]
        n99 = Negate(x=w713) -> (-x=w714:dbl)
        n100 = In Range and Coerce(upper limit=w713, x=w712, lower limit=w714) -> (coerced(x)=w711:dbl)  [unwired: 1 out]
      }
    }
    n101 = Build Array(w123, w122, w121, w120, w119) -> (w78:dbl[])
    n102 = Equal To 0?(x=w61) -> (x = 0?=w57:bool)
    n103 = case shown="3" "Fake pressure type" {
      tunnel: "Fake p.comp slider" -> [w269 w276 w280 _ w304]
      tunnel: [w267 w274 w283 w297 w307] -> w59
      tunnel: [w266 w273 w282 w300 w306] -> w58
      tunnel: w43 -> [w265 w272 w281 _ w305]
      tunnel: w57 -> [_ _ _ _ _]
      tunnel: w52 -> [_ _ _ w288 _]
      tunnel: [FALSE FALSE FALSE FALSE w303] -> w44
      frame 0, Default {
        w268 = FALSE ("Activate")
        n104 = Select(t=w269, s=w268, f=-1.0) -> (s? t:f=w266:dbl)
        n105 = Select(t=w269, s=w268, f=w265) -> (s? t:f=w267:dbl)
      }
      frame 1 {
        w275 = TRUE ("Activate")
        n106 = Select(t=w276, s=w275, f=-1.0) -> (s? t:f=w273:dbl)
        n107 = Select(t=w276, s=w275, f=w272) -> (s? t:f=w274:dbl)
      }
      frame 2 {
        n108 = Less?(x=w281, y=w280) -> (x < y?=w279:bool)
        n109 = Select(t=w280, s=w279, f=-2.0) -> (s? t:f=w282:dbl)
        n110 = Select(t=w280, s=w279, f=w281) -> (s? t:f=w283:dbl)
      }
      frame 3 {
        n111 = feedback #2() -> (w291:dbl)  [unwired: 1 in]
        n112 = Not(x="Start - Bosch Fake PB") -> (.not. x?=w292:bool)
        n113 = feedback-in #2(w288, w292) -> ()
        n114 = And(x="Start log with ramp 3", y="Start - Bosch Fake PB") -> (x .and. y?=w289:bool)
        n115 = Subtract(x=w288, y=w291) -> (x-y=w287:dbl)
        "Elapsed time 3" <- w287
        n116 = Greater?(x=w287, y=8.0) -> (0:w295:bool)
        n117 = shared-variable "NI-cRIO9022-0148F012\\Log variables.lvlib\\Start-log"(w289) -> ()  [unwired: 1 in, 1 out]
        n118 = And(x=w295, y="Start log with ramp 3") -> (x .and. y?=w294:bool)
        n119 = shared-variable "NI-cRIO9022-0148F012\\Log variables.lvlib\\Ramp_done"(w294) -> ()  [unwired: 1 in, 1 out]
        n120 = case shown="True" w295 {
          frame False {
          }
          frame True {
            n121 = property on="Start - Bosch Fake PB" class="Bool (strict)"("Value"=FALSE ("Start - Bosch array")) -> ()  [unwired: 2 in, 2 out]
          }
        }
        n122 = Interpolate 1D Array(1:w287, 2:"Bosch array 2") -> (0:w299:dbl)
        n123 = Select(t=w299, s="Start - Bosch Fake PB", f=4.0) -> (s? t:f=w297:dbl)
        n124 = Select(t=w297, s="Start - Bosch Fake PB", f=-3.0) -> (s? t:f=w300:dbl)
      }
      frame 4 {
        n125 = Less?(x=w305, y=w304) -> (x < y?=w303:bool)
        n126 = Select(t=w304, s=w303, f=-4.0) -> (s? t:f=w306:dbl)
        n127 = Select(t=w304, s=w303, f=w305) -> (s? t:f=w307:dbl)
      }
    }
    n128 = case shown="True" "Activate limits" {
      tunnel: w59 -> [w311 w320]
      tunnel: [w311 w319] -> w32
      tunnel: [w310 "Lower pressure limit [bar]"] -> w73
      tunnel: [w310 "Upper pressure limit [bar]"] -> w72
      tunnel: w43 -> [w309 w316]
      tunnel: [w309 w312] -> w41
      frame False {
        w310 = sgl 0.0 ("Lower pressure limit [bar]")
      }
      frame True {
        # "Pb fake with limits"
        # "Pb with limits"
        n129 = Greater?(x=w316, y="Lower pressure limit [bar]") -> (0:w318:bool)
        n130 = Greater?(x=w320, y="Lower pressure limit [bar]") -> (0:w323:bool)
        n131 = Select(t=w316, s=w318, f="Lower pressure limit [bar]") -> (s? t:f=w314:dbl)
        n132 = Less?(x=w314, y="Upper pressure limit [bar]") -> (x < y?=w317:bool)
        n133 = Select(t=w314, s=w317, f="Upper pressure limit [bar]") -> (s? t:f=w312:dbl)
        n134 = Select(t=w320, s=w323, f="Lower pressure limit [bar]") -> (s? t:f=w321:dbl)
        n135 = Less?(x=w321, y="Upper pressure limit [bar]") -> (x < y?=w322:bool)
        n136 = Select(t=w321, s=w322, f="Upper pressure limit [bar]") -> (s? t:f=w319:dbl)
      }
    }
    n137 = Build Array("dL HP cutoff freq [Hz]", "dL lowpass cutoff freq [Hz]", "Pb highpass cutoff freq [Hz]", "Pb lowpass cutoff freq [Hz]", w73, w72) -> (w70:dbl[])
    n138 = call <vilib>:"Butterworth Filter PtByPt.vi"("initialize"="Initialise Pb lowpass filter", "order"=1, "filter type"=Filter_Passband_Type."Lowpass", "low cutoff freq: fl"="Pb lowpass cutoff freq [Hz]", "sampling freq: fs"=w104, "x"=w32) -> ("Filtered x"=w50:dbl)  [unwired: 3 in, 1 out]
    "P.B.LP" <- w50
    n139 = Multiply(x=w37, y=w32) -> (x*y=w36:dbl)
    n140 = Add(x=w39, y=w36) -> (x+y=w27:dbl)
    n141 = Build Array(w146, w27) -> (w103:dbl[])
    n142 = Build Array (concatenate)(w50, w102, w103) -> (w83:dbl[])
    n143 = Or(x=w44, y="Bypass low-pass filter") -> (x .or. y?=w46:bool)
    n144 = Build Array (concatenate)(w52, w94, w83, w82) -> (w91:dbl[])
    n145 = case shown="True" w46 {
      tunnel: [w261 w263] -> w51
      tunnel: w50 -> [w261 _]
      tunnel: w41 -> [_ w263]
      tunnel: [1.0 ("t") 0.0 ("t")] -> w47
      frame False {
      }
      frame True {
      }
    }
    n146 = Delete From Array(array=w91, length=1, index=0) -> (array with subset deleted=w90:dbl[])  [unwired: 1 out]
    n147 = case shown="2" "Bosch input type" {
      tunnel: ["Bosch valve, voltage" w358 w389] -> w87
      tunnel: w51 -> [_ _ w377]
      tunnel: w101 -> [_ _ w388]
      tunnel: [w346 w352 w383] -> w63
      tunnel: [w346 w352 "dpOpen (bar)"] -> w68
      tunnel: [w346 w352 w374] -> w67
      tunnel: [w346 w352 w373] -> w66
      tunnel: [w346 w352 w372] -> w65
      tunnel: [dbl[] [0.0, 0.0, 0.0] ("Separate output") dbl[] [0.0, 0.0, 0.0] ("Separate output") w370] -> w49
      tunnel: w52 -> [_ w362 _]
      tunnel: [0.0 0.0 w379] -> w48
      frame 0, Default {
        w346 = 0.0 ("f")
        # "Manual control, Bosch valve"
        n148 = case shown="True" "Reset Bosch" {
          frame False {
          }
          frame True {
            n149 = property on="Bosch valve, voltage" class="Slide (strict)"("Value"=0.0 ("t")) -> ()  [unwired: 2 in, 2 out]
          }
        }
      }
      frame 1 {
        w352 = -1.0 ("f")
        n150 = And(x="Start log with ramp 2", y="Start - Bosch array") -> (x .and. y?=w357:bool)
        n151 = feedback #3() -> (w365:dbl)  [unwired: 1 in]
        n152 = Not(x="Start - Bosch array") -> (.not. x?=w366:bool)
        n153 = feedback-in #3(w362, w366) -> ()
        n154 = shared-variable "NI-cRIO9022-0148F012\\Log variables.lvlib\\Start-log"(w357) -> ()  [unwired: 1 in, 1 out]
        n155 = Subtract(x=w362, y=w365) -> (x-y=w360:dbl)
        "Elapsed time 2" <- w360
        n156 = Greater?(x=w360, y=32.0) -> (0:w353:bool)
        n157 = And(x=w353, y="Start log with ramp 2") -> (x .and. y?=w354:bool)
        n158 = Interpolate 1D Array(1:w360, 2:"Bosch array") -> (0:w363:dbl)
        n159 = case shown="True" w353 {
          frame False {
          }
          frame True {
            n160 = property on="Start - Bosch array" class="Bool (strict)"("Value"=FALSE ("Start - Bosch array")) -> ()  [unwired: 2 in, 2 out]
          }
        }
        n161 = shared-variable "NI-cRIO9022-0148F012\\Log variables.lvlib\\Ramp_done"(w354) -> ()  [unwired: 1 in, 1 out]
        n162 = Select(t=w363, s="Start - Bosch array", f=0.0) -> (s? t:f=w358:dbl)
      }
      frame 2 {
        # "To log"
        # "PID, Bosch valve"
        # "Control system, Bosch valve"
        n163 = Select(t="Bosch valve, pressure", s="Operation mode", f=w377) -> (s? t:f=w382:dbl)
        n164 = Select(t="Bosch valve, pressure", s="Operation mode", f=-1.0) -> (s? t:f=w383:dbl)
        n165 = case shown="0, Default" "Controller selection" {
          tunnel: ["Proportional Gain" "Proportional Gain 2"] -> w374
          tunnel: ["Integral Gain" "Integral Gain 2"] -> w373
          tunnel: ["Derivative Gain" "Derivative Gain 2"] -> w372
          frame 0, Default {
          }
          frame 1 {
          }
        }
        n166 = Subtract(x=w382, y=w388) -> (x-y=w392:dbl)
        n167 = case shown="True" "Feed forward activate" {
          tunnel: w382 -> [_ w673]
          tunnel: [0.0 w672] -> w379
          frame False {
          }
          frame True {
            n168 = Interpolate 1D Array(1:w673, 2:"Bosch mapping 180bar - opening based") -> (0:w672:dbl)
          }
        }
        n169 = To Double Precision Float(number=w392) -> (double precision float=w375:dbl)
        n170 = xnode "PID (Parallel) with monitoring.vi"("Error"=w375, "Proportional Gain"=w374, "Integral Gain"=w373, "Derivative Gain"=w372, "Initialize"="Initialize bosch") -> ("Separate output"=w370:dbl[], "Output"=w369:dbl)  [unwired: 1 in, 10 out]
        n171 = Add(x=w379, y=w369) -> (x+y=w378:dbl)
        n172 = case shown="True" "Reset Bosch 2" {
          frame False {
          }
          frame True {
            n173 = property on="Bosch valve, pressure" class="Slide (strict)"("Value"=0.0 ("Bosch valve, pressure")) -> ()  [unwired: 2 in, 2 out]
          }
        }
        n174 = Select(t=w378, s="Run Bosch control system", f=sgl 0.0) -> (s? t:f=w389:dbl)
      }
    }
    n175 = Build Array(w58, w63) -> (w62:dbl[])
    n176 = case shown="True" "Activate comp" {
      tunnel: [w326 w333] -> w126
      tunnel: w61 -> [w326 w332]
      tunnel: [0.0 ("upper limit") w331] -> w125
      tunnel: w102 -> [_ w329]
      tunnel: [w324 "Comp.Q.to.U.gain"] -> w89
      tunnel: [w324 "Comp.kF.gain"] -> w88
      frame False {
        w324 = 0.0 ("Q_to_U_gain")
      }
      frame True {
        n177 = Multiply(x=w329, y="Comp.kF.gain") -> (x*y=w340:dbl)
        n178 = Multiply(x=w340, y="Comp.Q.to.U.gain") -> (x*y=w337:dbl)
        n179 = Equal?(x=w332, y=sgl 0.0) -> (x = y?=w335:bool)
        n180 = In Range and Coerce(upper limit=1.0, x=w337, lower limit=-1.0) -> (coerced(x)=w334:dbl)  [unwired: 1 out]
        n181 = Select(t=0.0, s=w335, f=w334) -> (s? t:f=w331:dbl)
        "u_DCV_comp" <- w331
        n182 = Subtract(x=w332, y=w331) -> (x-y=w333:dbl)
      }
    }
    "u_DCV" <- w126
    n183 = Build Array(w47, w68, w67, w66, w65) -> (w64:dbl[])
    n184 = Build Array(w88, w89) -> (w77:dbl[])
    n185 = In Range and Coerce(upper limit=sgl 1.0, x=w87, lower limit=sgl 0.0) -> (coerced(x)=w124:dbl)  [unwired: 1 out]
    "u_Bosch" <- w124
    n186 = Build Array(w126, w125, w124) -> (w100:dbl[])
    n187 = case shown="0, Default" "DCV Output" {
      tunnel: [w341 0.0 ("t")] -> w135
      tunnel: w126 -> [w341 w344]
      tunnel: [0.0 ("t") w344] -> w134
      frame 0, Default {
      }
      frame 1 {
      }
    }
    n188 = Select(t=w124, s="Activate Bosch", f=sgl 0.0 ("t")) -> (s? t:f=w217:dbl)
    n189 = call "Anti_deadband_PVG.vi"("x"=w135) -> ("y"=w185:sgl)
    n190 = Multiply(x=w185, y=sgl 3.0) -> (x*y=w251:sgl)
    n191 = Multiply(x=w217, y=sgl 10.0) -> (x*y=w127:dbl)
    "U_Bosch" <- w127
    n192 = call "Anti_deadband_Hawe.vi"("x"=w134) -> ("y"=w190:sgl)
    n193 = Add(x=w251, y=sgl 6.0) -> (x+y=w137:sgl)
    n194 = Multiply(x=w190, y=sgl 10.0) -> (x*y=w216:sgl)
    n195 = Select(t=w137, s="Activate DCV", f=sgl 6.0) -> (s? t:f=w128:sgl)
    "U_PVG" <- w128
    n196 = Select(t=w216, s="Activate DCV", f=sgl 0.0) -> (s? t:f=w129:sgl)
    "U_Hawe" <- w129
    n197 = Build Array(w129, w128, w127) -> (w99:dbl[])
    n198 = xnode "Butterworth Coefficients"("cutoff frequency (Hz)"="cutoff frequency (Hz) pressures", "sample rate (S/s)"="sample rate (S/s) pressures") -> ("scaled coefficients"=w209:i32[])  [unwired: 1 in, 1 out]
    n199 = xnode "Butterworth Coefficients"("cutoff frequency (Hz)"="cutoff frequency (Hz)l_cyl", "sample rate (S/s)"="sample rate (S/s) l_cyl") -> ("scaled coefficients"=w208:i32[])  [unwired: 1 in, 1 out]
    n200 = xnode "Butterworth Coefficients"("cutoff frequency (Hz)"="cutoff frequency (Hz) Q", "sample rate (S/s)"="sample rate (S/s) Q") -> ("scaled coefficients"=w199:i32[])  [unwired: 1 in, 1 out]
    n201 = xnode "Butterworth Coefficients"("cutoff frequency (Hz)"="cutoff frequency (Hz) FB_PVG", "sample rate (S/s)"="sample rate (S/s) FB_PVG") -> ("scaled coefficients"=w198:i32[])  [unwired: 1 in, 1 out]
    n202 = xnode "Butterworth Coefficients"("cutoff frequency (Hz)"="cutoff frequency (Hz) FB_Bosch", "sample rate (S/s)"="sample rate (S/s) FB_Bosch") -> ("scaled coefficients"=w197:i32[])  [unwired: 1 in, 1 out]
    n203 = xnode "Butterworth Coefficients"("cutoff frequency (Hz)"="cutoff frequency (Hz) FB_Hawe", "sample rate (S/s)"="sample rate (S/s) FB_Hawe") -> ("scaled coefficients"=w196:i32[])  [unwired: 1 in, 1 out]
    n204 = xnode "Butterworth Coefficients"("cutoff frequency (Hz)"="cutoff frequency (Hz) Strain", "sample rate (S/s)"="sample rate (S/s) Strain") -> ()  [unwired: 1 in, 2 out]
    n205 = Build Array (concatenate)(w52, w90, w100, w99, w62, w49, w48, w20) -> (w98:dbl[])
    n206 = shared-variable "NI-cRIO9022-0148F012\\Log variables.lvlib\\Active-log"() -> (→"Active.log":bool)  [unwired: 1 in, 1 out]
    n207 = Build Array (concatenate)(w52, w78, w77, w70, w64) -> (w69:dbl[])
    n208 = shared-variable "NI-cRIO9022-0148F012\\Log variables.lvlib\\Start-log"("Start.log") -> ()  [unwired: 1 in, 1 out]
    n209 = xnode "Read/Write Control"("FPGA VI Reference In"=w173, "error in"=w172, "S_Bosch"=w127, "S_Hawe"=w129, "S_PVG"=w128, "FPGA_filter_dt(uSec)"="FPGA_dt(uSec)", "filter_coeff_pressures"=w209, "filter_coeff_l_cyl"=w208, "filter_coeff_Q"=w199, "filter_coeff_FB_PVG"=w198, "filter_coeff_Bosch"=w197, "filter_coeff_Hawe"=w196, "Excitation Voltage Strain Gauge"="Excitation Voltage Strain Gauge", "Data Rate Strain Gauge"="Data Rate Strain Gauge") -> ("FPGA VI Reference Out"=w171:refnum<k20>, "error out"=w170:errorcluster)
    n210 = shared-variable "NI-cRIO9022-0148F012\\TCPIP_Variables.lvlib\\Rio-to-pc-fixed-values"(w69) -> ()  [unwired: 1 in, 1 out]
    n211 = shared-variable "NI-cRIO9022-0148F012\\TCPIP_Variables.lvlib\\Rio-to-pc-1"(w98) -> ()  [unwired: 1 in, 1 out]
    n212 = Tick Count (ms)() -> (millisecond timer value=w164:u32)
    n213 = node-c288() -> ()  [unwired: 1 in, 1 out]
  }
  n214 = node-c288(w8) -> ()  [unwired: 7 out]
  n215 = xnode "Close FPGA VI Reference"("FPGA VI Reference In"=w5, "error in"=w4) -> ()  [unwired: 1 out]
